vi "dfd_FXP PtByPt Direct IIR I Transposed.vi"(0 "x":T2={"value"=0, "wl"=0, "iwl"=0, "Signed"=TRUE} {"value" format="%.0x"}, 1 "coef b[0..M]":T1, 2 "coef a[1..N]":T1, 5 "filtering statistics in":T5(array[cluster]) {"statistics information"."min value" format="%.2f"; "statistics information"."max value" format="%.2f"; "Quantizer Source" items=["Coefficients a/k"=0, "Coefficients b/v"=7, "Input"=1, "Output"=2, "Multiplicand"=3, "Product"=4, "Sum"=5, "Delay"=6]}, 6 "quantizers":T6[](array[typedef]) {"source" items=["Coef a/k"=0, "Coef b/v"=7, "Input"=1, "Output"=2, "Multiplicand"=3, "Product"=4, "Sum"=5, "Delay"=6, "Gain"=8]}, 7 "xState in":i64[](array[numeric]), 9 "yState in":i64[](array[numeric])) -> (11 "yState out":i64[](array[numeric]), 13 "xState out":i64[](array[numeric]), 14 "filtered x":T2={"value"=0, "wl"=0, "iwl"=0, "Signed"=TRUE} {"value" format="%.0x"}, 19 "filtering statistics out":T5(array[cluster]) {"statistics information"."min value" format="%.2f"; "statistics information"."max value" format="%.2f"; "Quantizer Source" items=["Coefficients a/k"=0, "Coefficients b/v"=7, "Input"=1, "Output"=2, "Multiplicand"=3, "Product"=4, "Sum"=5, "Delay"=6]})   [LabVIEW 2017, in "NI_DigFilter_FXP.lvlib"]
uses:
  <vilib>/addons/Digital Filter Design/NI_DigFilter_FXP.lvlib
  <vilib>/addons/Digital Filter Design/_Objects.llb/dfd_DFXP Data Type (scaler).ctl
  <vilib>/addons/Digital Filter Design/_Objects.llb/dfd_DFXP Operation Parameter.ctl
  <vilib>/addons/Digital Filter Design/_Objects.llb/dfd_Internal Quantization Srcs.ctl
  <vilib>/addons/Digital Filter Design/_Objects.llb/dfd_DFXP Data Type (vector).ctl
  <vilib>/addons/Digital Filter Design/_Objects.llb/DFD Quantization Sources.ctl
  <vilib>/addons/Digital Filter Design/_Objects.llb/DFD FXP Statistics Data.ctl
  <vilib>/addons/Digital Filter Design/NI_DigFilterLicensed.lvlib
panel:
  in  "states":T1
  in  "state":T2={"value"=0, "wl"=0, "iwl"=0, "Signed"=TRUE} {"value" format="%.0x"}
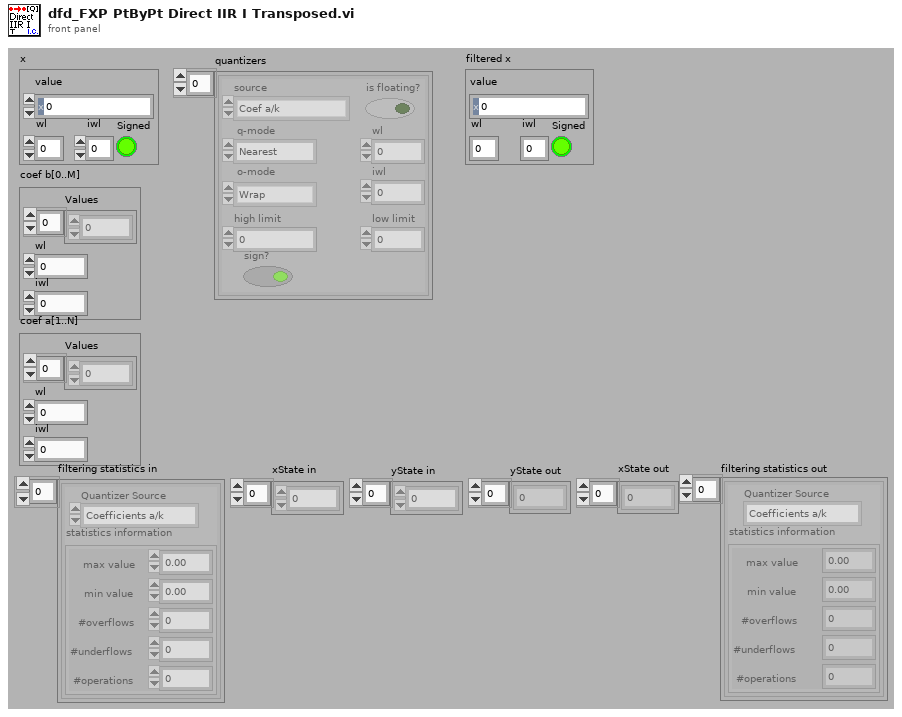
[diagram p1: front panel]
types:
  T1 = typedef "dfd_DFXP Data Type (vector).ctl" = cluster{"Values":i64[], "wl":i16, "iwl":i16}
  T2 = typedef "dfd_DFXP Data Type (scaler).ctl" = cluster{"value":i64, "wl":i16, "iwl":i16, "Signed":bool}
  T3 = typedef "NI_DigFilterLicensed.lvlib/DFD Quantization Sources.ctl" = u16
  T4 = typedef "NI_DigFilterLicensed.lvlib/DFD FXP Statistics Data.ctl" = cluster{"max value":ext, "min value":ext, "#overflows":i32, "#underflows":i32, "#operations":i32}
  T5 = cluster{"Quantizer Source":T3, "statistics information":T4}[]
  T6 = typedef "dfd_DFXP Operation Parameter.ctl" = cluster{"source":T7, "is floating?":bool, "o-mode":enum16{"Saturation", "Wrap"}, "q-mode":enum16{"Nearest", "Truncation"}, "wl":i16, "high limit":i64, "low limit":i64, "iwl":i16, "sign?":bool}
  T7 = typedef "NI_DigFilterLicensed.lvlib/dfd_Internal Quantization Srcs.ctl" = u16
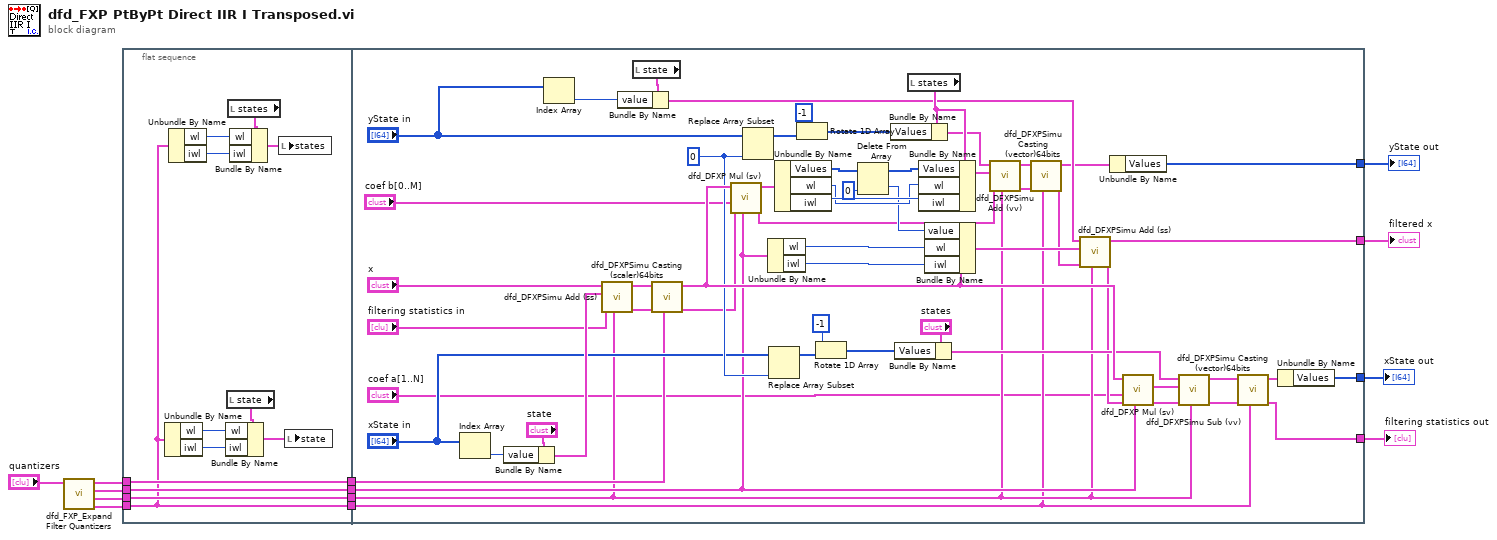
[diagram p0: block diagram]
diagram:
  n1 = call <vilib>:"dfd_FXP_Expand Filter Quantizers.vi"("FXPOPs"="quantizers") -> ("Delay"=w10:T6, "Sum"=w11:T6, "Product"=w12:T6, "Multiplicand"=w4:T6)  [unwired: 7 out]
  n2 = flat-sequence {
    tunnel: w10 -> [w16]
    tunnel: w4 -> [w21]
    tunnel: w12 -> [w20]
    tunnel: w11 -> [w19]
    tunnel: [w21] -> w9
    tunnel: [w20] -> w8
    tunnel: [w19] -> w7
    tunnel: [w16] -> w6
    tunnel: w9 -> [w35]
    tunnel: w8 -> [w34]
    tunnel: w7 -> [w33]
    tunnel: w6 -> [w32]
    tunnel: [w31] -> w5
    tunnel: [w30] -> w3
    tunnel: [w29] -> w2
    tunnel: [w28] -> w1
    frame #0 {
      n3 = Unbundle By Name(w16) -> ("wl"=w24:i16, "iwl"=w23:i16)
      n4 = Unbundle By Name(w16) -> ("wl"=w17:i16, "iwl"=w18:i16)
      n5 = local read "state"() -> (w25:T2)
      n6 = Bundle By Name(cluster=w25, "wl"=w24, "iwl"=w23) -> (w22:T2)
      n7 = local read "states"() -> (w14:T1)
      n8 = Bundle By Name(cluster=w14, "wl"=w17, "iwl"=w18) -> (w15:T1)
      n9 = local write "states"(w15) -> ()
      n10 = local write "state"(w22) -> ()
    }
    frame #1 {
      w67 = i64 0 ("Bits pattern")
      n11 = Index Array(array="xState in") -> (element=w41:i64)  [unwired: 1 in]
      n12 = Bundle By Name(cluster="state", "value"=w41) -> (w63:T2)
      n13 = Index Array(array="yState in") -> (element=w54:i64)  [unwired: 1 in]
      n14 = call <vilib>:"dfd_DFXPSimu Add (ss).vi"("op params"=w33, "filtering statistics in"="filtering statistics in", "value in 2"=w63, "value in 1"="x") -> ("filtering statistics out"=w45:T5, "value out"=w44:T2)  [unwired: 1 in, 5 out]
      n15 = local read "state"() -> (w66:T2)
      n16 = Bundle By Name(cluster=w66, "value"=w54) -> (w65:T2)
      n17 = call <vilib>:"dfd_DFXPSimu Casting (scaler)64bits.vi"("op params"=w35, "filtering statistics in"=w45, "Value in"=w44) -> ("filtering statistics out"=w46:T5, "Value out"=w80:T2)  [unwired: 2 in, 5 out]
      n18 = call <vilib>:"dfd_DFXP Mul (sv).vi"("op params"=w34, "filtering statistics in"=w46, "Value in 2"="coef b[0..M]", "Value in"=w80) -> ("filtering statistics out"=w50:T5, "Value out"=w68:T1)  [unwired: 1 in, 5 out]
      n19 = Replace Array Subset(array="yState in", new element=w67) -> (w39:i64[])  [unwired: 1 in]
      n20 = Unbundle By Name(w34) -> ("wl"=w81:i16, "iwl"=w82:i16)
      n21 = Replace Array Subset(array="xState in", new element=w67) -> (w43:i64[])  [unwired: 1 in]
      n22 = Unbundle By Name(w68) -> ("Values"=w69:i64[], "wl"=w77:i16, "iwl"=w78:i16)
      n23 = Rotate 1D Array(1:w39, 2:-1 ("n")) -> (0:w70:i64[])
      n24 = Rotate 1D Array(1:w43, 2:-1 ("n")) -> (0:w55:i64[])
      n25 = Delete From Array(array=w69, index=0) -> (deleted portion=w62:i64, array with subset deleted=w61:i64[])  [unwired: 1 in]
      n26 = Bundle By Name(cluster="states", "Values"=w55) -> (w72:T1)
      n27 = local read "states"() -> (w76:T1)
      n28 = Bundle By Name(cluster=w76, "Values"=w70) -> (w74:T1)
      n29 = Bundle By Name(cluster=w76, "Values"=w61, "wl"=w77, "iwl"=w78) -> (w75:T1)
      n30 = Bundle By Name(cluster=w80, "value"=w62, "wl"=w81, "iwl"=w82) -> (w79:T2)
      n31 = call <vilib>:"dfd_DFXPSimu Add (vv).vi"("op params"=w33, "filtering statistics in"=w50, "values in 2"=w75, "values in 1"=w74) -> ("filtering statistics out"=w51:T5, "values out"=w49:T1)  [unwired: 6 out]
      n32 = call <vilib>:"dfd_DFXPSimu Casting (vector)64bits.vi"("op params"=w32, "filtering statistics in"=w51, "Value in"=w49) -> ("filtering statistics out"=w53:T5, "Value out"=w52:T1)  [unwired: 1 in, 6 out]
      n33 = call <vilib>:"dfd_DFXPSimu Add (ss).vi"("op params"=w33, "filtering statistics in"=w53, "value in 2"=w79, "value in 1"=w65) -> ("filtering statistics out"=w59:T5, "value out"=w29:T2)  [unwired: 6 out]
      n34 = Unbundle By Name(w52) -> ("Values"=w30:i64[])
      n35 = call <vilib>:"dfd_DFXP Mul (sv).vi"("op params"=w34, "filtering statistics in"=w59, "Value in 2"="coef a[1..N]", "Value in"=w80) -> ("filtering statistics out"=w60:T5, "Value out"=w71:T1)  [unwired: 1 in, 5 out]
      n36 = call <vilib>:"dfd_DFXPSimu Sub (vv).vi"("op params"=w33, "filtering statistics in"=w60, "values in 2"=w71, "values in 1"=w72) -> ("filtering statistics out"=w58:T5, "values out"=w56:T1)  [unwired: 6 out]
      n37 = call <vilib>:"dfd_DFXPSimu Casting (vector)64bits.vi"("op params"=w32, "filtering statistics in"=w58, "Value in"=w56) -> ("filtering statistics out"=w28:T5, "Value out"=w57:T1)  [unwired: 1 in, 6 out]
      n38 = Unbundle By Name(w57) -> ("Values"=w31:i64[])
    }
  }
  "yState out" <- w3
  "filtered x" <- w2
  "xState out" <- w5
  "filtering statistics out" <- w1
